vi "Compute Expected DAQ Loop Interval.vi"(7 "Measurement config":T1={"Data Rate 9775"=1000000.0, "Data Rate 9215"=20000.0, "Samples RMS 9215"=1000, "Samples RMS 9775"=1000}, 8 "error in (no error)":errorcluster, 9 "MinDemoWait (20ms)":u32=20, 10 "MaxDemoWait (10000)":u32=10000, 11 "DemoMode":bool) -> (0 "error out":errorcluster, 1 "WaitFunction Value":u32, 2 "Computed Loop Interval":u32)   [LabVIEW 2019, in "DAQ_Engine.lvclass"]
doc: "Developed by Kevin Thompson\nkevin@thompsonengineering.net\n\nCopyright 2020\nThompson Engineering, LLC"
uses:
  DAQ_Engine.lvclass
  Common/DataTypes/Measurement Config--cluster.ctl
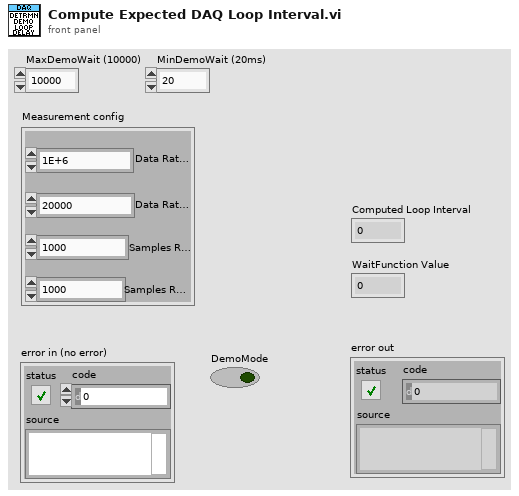
[diagram p1: front panel]
types:
  T1 = typedef "Measurement Config--cluster.ctl" = cluster{"Data Rate 9775":dbl, "Data Rate 9215":dbl, "Samples RMS 9215":u32, "Samples RMS 9775":u32}
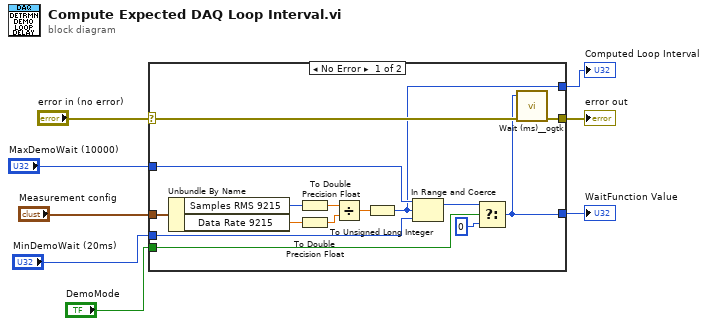
[diagram p0: block diagram]
diagram:
  n1 = case shown="No Error" "error in (no error)" {
    selector: "error in (no error)" -> [w14 w24]
    tunnel: [w19 w24] -> w8
    tunnel: "Measurement config" -> [w18 _]
    tunnel: "DemoMode" -> [w15 _]
    tunnel: "MaxDemoWait (10000)" -> [w13 _]
    tunnel: "MinDemoWait (20ms)" -> [w12 _]
    tunnel: [w10 _] -> w2
    tunnel: [w9 _] -> w1
    frame No Error {
      n2 = Unbundle By Name(w18) -> ("Samples RMS 9215"=w17:u32, "Data Rate 9215"=w20:dbl)
      n3 = To Double Precision Float(number=w17) -> (double precision float=w22:dbl)
      n4 = To Double Precision Float(number=w20) -> (double precision float=w21:dbl)
      n5 = Divide(x=w22, y=w21) -> (x/y=w23:dbl)
      n6 = To Unsigned Long Integer(number=w23) -> (unsigned 32bit integer=w10:u32)
      n7 = In Range and Coerce(upper limit=w13, x=w10, lower limit=w12) -> (coerced(x)=w11:u32)  [unwired: 1 out]
      n8 = Select(t=w11, s=w15, f=u32 0) -> (s? t:f=w9:u32)
      n9 = call <userlib>:"Wait (ms)__ogtk.vi"("error in (no error)"=w14, "milliseconds to wait"=w9) -> ("error out"=w19:errorcluster)  [unwired: 8 in, 1 out]
    }
    frame Error {
    }
  }
  "error out" <- w8
  "Computed Loop Interval" <- w2
  "WaitFunction Value" <- w1
